vi "Get Current Temperature.vi"(8 "error in (no error)":cluster{"状态":bool, "代码":i32, "源":string} caption="错误输入（无错误）", 11 "硬件蒸发冷却器输入":refnum<class "HW Evaporative Cooler.lvclass">) -> (0 "error out":cluster{"状态":bool, "代码":i32, "源":string} caption="错误输出", 2 "水位":dbl)   [LabVIEW 2013, in "HW Evaporative Cooler.lvclass"]
doc: "该VI设定水位控制器负责监控的变量。该VI被调用时将返回变量的当前值。"
uses:
  HW Evaporative Cooler.lvclass
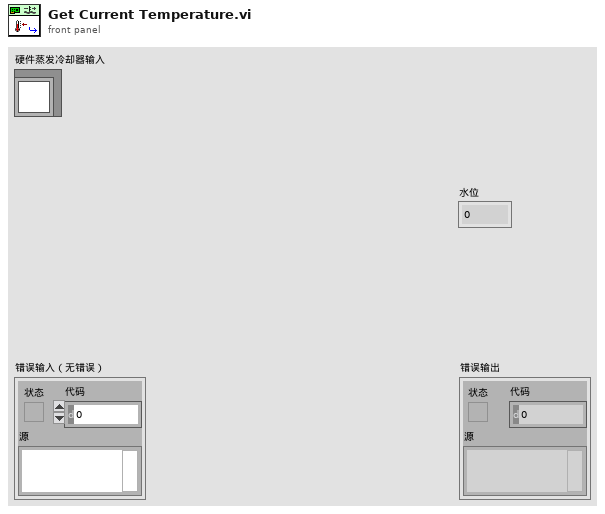
[diagram p1: front panel]
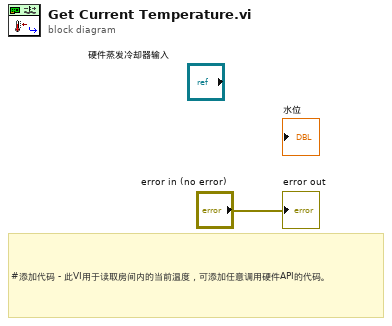
[diagram p0: block diagram]
diagram:
  # "#添加代码 - 此VI用于读取房间内的当前温度，可添加任意调用硬件API的代码。"
  "error out" <- "error in (no error)"
